vi "Testing UDP Discover.vi"() -> ()   [LabVIEW 2020]
uses:
  <vilib>/Utility/tcp.llb/UDP Multicast Read-Write Open.vi
panel:
  out "name 2":string
  out "name":string
  out "address":u32
  out "data out 3":string
  out "data out 2":string
  out "data out":string
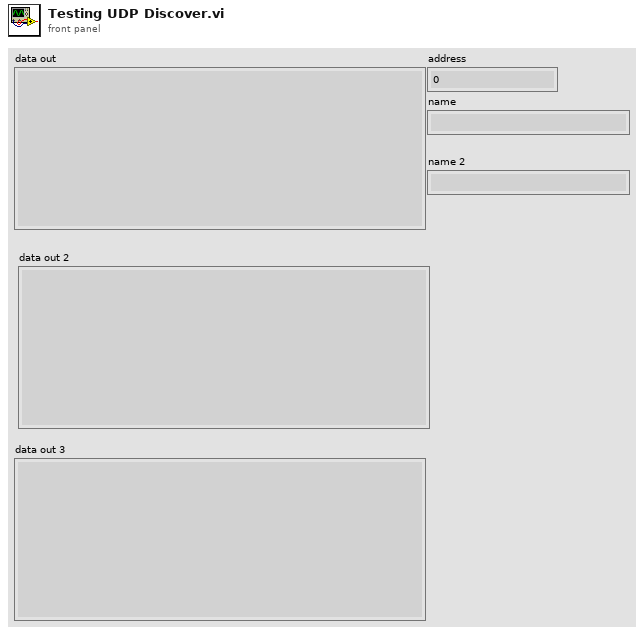
[diagram p1: front panel]
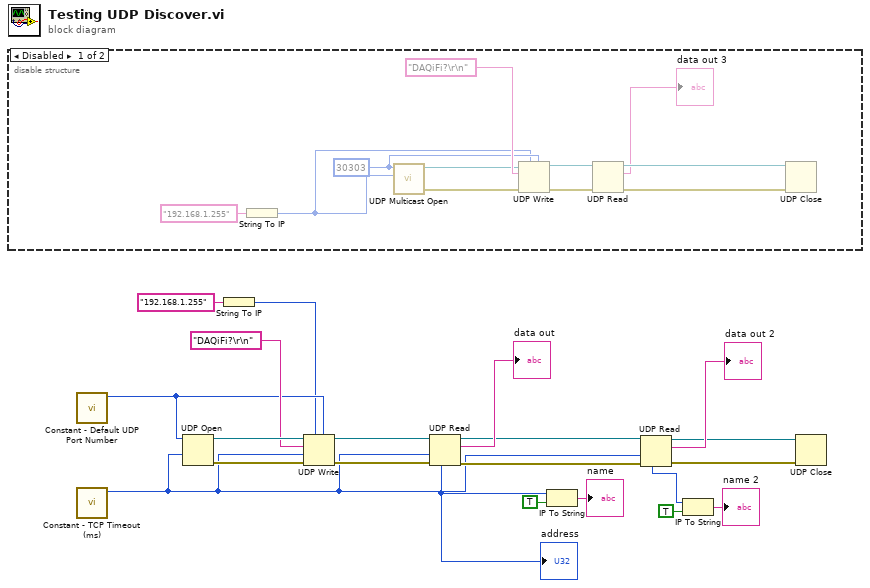
[diagram p0: block diagram]
diagram:
  n1 = disable-structure shown="Disabled" {
    frame Disabled {
      w23 = u16 30303 ("port")
      n2 = String To IP(1:"192.168.1.255" ("name")) -> (0:w22:u32)
      n3 = call-poly <vilib>:"UDP Multicast Open.vi"("multicast addr"=w22, "port"=w23) -> ("error out"=w29:errorcluster, "connection ID"=w30:refnum<k16>)  [unwired: 7 in, 1 out]
      n4 = UDP Write(address=w22, port or service name=w23, connection ID=w30, data in="DAQiFi?\r\n", 8:w29) -> (error out=w25:errorcluster, 3:w28:refnum<k16>)  [unwired: 1 in]
      n5 = UDP Read(connection ID=w28, 8:w25) -> (data out=→"data out 3":string, error out=w26:errorcluster, 3:w27:refnum<k16>)  [unwired: 2 in, 2 out]
      n6 = UDP Close(connection ID=w27, 8:w26) -> ()  [unwired: 2 out]
    }
    frame Enabled {
    }
  }
  n7 = call "Constant - Default UDP Port Number.vi"() -> ("port"=w15:u16)  [unwired: 11 in]
  n8 = call "Constant - TCP Timeout (ms).vi"() -> ("timeout (ms)"=w9:i32)  [unwired: 11 in]
  n9 = UDP Open(9:w9, 11:w15) -> (port=w21:refnum<k16>, 0:w18:errorcluster)  [unwired: 3 in, 1 out]
  n10 = String To IP(1:"192.168.1.255" ("name")) -> (0:w7:u32)
  n11 = UDP Write(address=w7, port or service name=w15, connection ID=w21, data in="DAQiFi?\r\n", 8:w18, 9:w9) -> (error out=w19:errorcluster, 3:w20:refnum<k16>)
  n12 = UDP Read(connection ID=w20, timeout ms (25000)=w9, 8:w19) -> (data out=→"data out":string, error out=w10:errorcluster, 3:w13:refnum<k16>, 6:w6:u32)  [unwired: 1 in, 1 out]
  "address" <- w6
  n13 = IP To String(1:TRUE ("dot notation? (F)"), 2:w6) -> (0:→"name":string)
  n14 = UDP Read(connection ID=w13, timeout ms (25000)=w9, 8:w10) -> (data out=→"data out 2":string, error out=w11:errorcluster, 3:w12:refnum<k16>, 6:w1:u32)  [unwired: 1 in, 1 out]
  n15 = IP To String(1:TRUE ("dot notation? (F)"), 2:w1) -> (0:→"name 2":string)
  n16 = UDP Close(connection ID=w12, 8:w11) -> ()  [unwired: 2 out]
